vi "AuMT8852B AFH EUT Report Rate.vi"(5 "EUT Reporting Rate (1)":i8=1 min=1 max=30, 7 "Set/Get (Set)":enum16{"Set", "Get"}(ring)=enum."Get", 8 "error in (no error)":errorcluster, 11 "VISA session":refnum<visa-resource-name>) -> (0 "error out":errorcluster, 2 "error code":i32, 3 "VISA session out":refnum<visa-resource-name>, 4 "EUT Reporting Rate out":i8=1 min=1 max=30)   [LabVIEW 2017]
doc: "Anritsu MT8852B Bluetooth Tester\n\nControls the rate, in seconds, at which the EUT generates local assessment reports.\n\nINPUTS\nSet/Get - whether the value is being sent to or retrieved from the instrument.\nEUT Reporting Rate - the rate (1-30 seconds) at which reports are generated.\n\nOUTPUTS\nEUT Reporting Rate out - the current rate at which reports are currently generated."
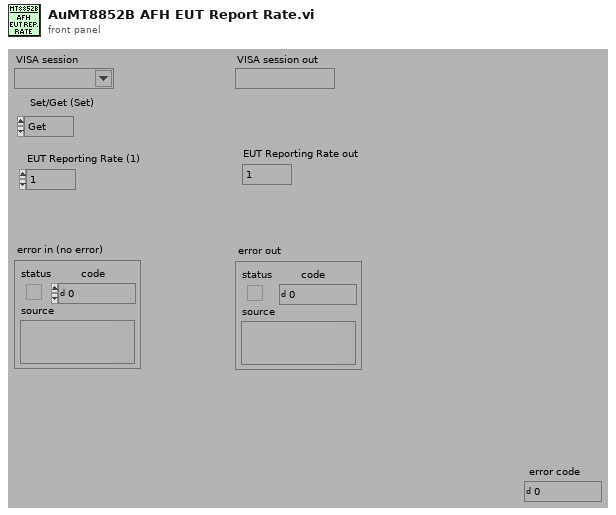
[diagram p1: front panel]
types:
  T1 = enum16{"Simulate", "Range check", "Cache", "Query instrument status"}
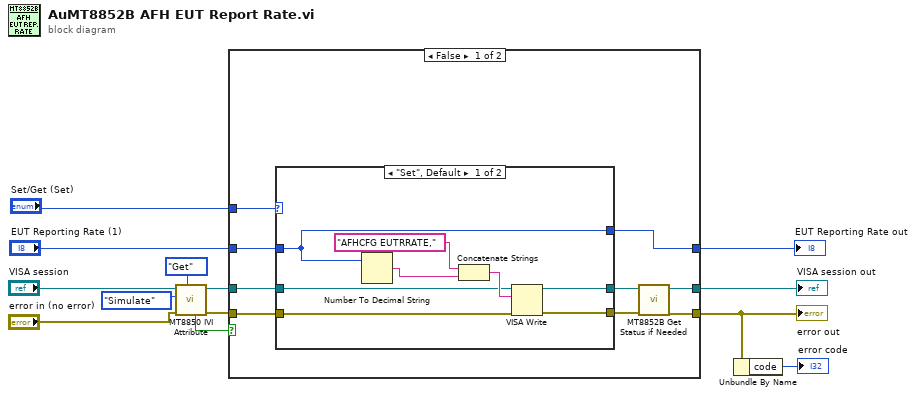
[diagram p0: block diagram]
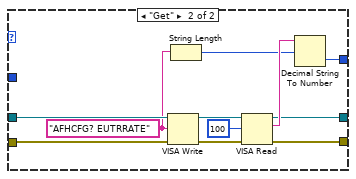
[diagram p2: hidden frame]
diagram:
  n1 = call <instrlib>:"MT8850 IVI Attribute.vi"("Set/Get (Set)"=enum16{"Set", "Get"}."Get", "error in (no error)"="error in (no error)", "Flag (Simulate)"=T1."Simulate", "VISA session"="VISA session") -> ("error out"=w12:errorcluster, "VISA session out"=w13:refnum<visa-resource-name>, "Value out"=w9:bool)  [unwired: 5 in]
  n2 = case shown="False" w9 {
    tunnel: [w18 w44] -> w7
    tunnel: [w19 w43] -> w6
    tunnel: w13 -> [w20 w44]
    tunnel: w12 -> [w21 w43]
    tunnel: [w22 w42] -> w3
    tunnel: "EUT Reporting Rate (1)" -> [w15 w42]
    tunnel: "Set/Get (Set)" -> [w14 _]
    frame False {
      n3 = case shown="\"Set\", Default" w14 {
        tunnel: w15 -> [w24 _]
        tunnel: [w24 w37] -> w22
        tunnel: [w25 w34] -> w16
        tunnel: [w26 w33] -> w17
        tunnel: w21 -> [w28 w36]
        tunnel: w20 -> [w27 w35]
        frame "Set", Default {
          n4 = Number To Decimal String(number=w24) -> (decimal integer string=w23:string)  [unwired: 1 in]
          n5 = Concatenate Strings("AFHCFG EUTRRATE," ("write buffer (\"\")"), w23) -> (w29:string)
          n6 = VISA Write(VISA resource name=w27, write buffer=w29, error in (no error)=w28) -> (VISA resource name out=w26:refnum<visa-resource-name>, error out=w25:errorcluster)  [unwired: 1 out]
        }
        frame "Get" {
          w32 = "AFHCFG? EUTRRATE" ("write buffer (\"\")")
          n7 = VISA Write(VISA resource name=w35, write buffer=w32, error in (no error)=w36) -> (VISA resource name out=w40:refnum<visa-resource-name>, error out=w41:errorcluster)  [unwired: 1 out]
          n8 = String Length(string=w32) -> (length=w31:i32)
          n9 = VISA Read(VISA resource name=w40, byte count=u32 100 ("byte count (0)"), error in (no error)=w41) -> (VISA resource name out=w33:refnum<visa-resource-name>, read buffer=w38:string, error out=w34:errorcluster)  [unwired: 1 out]
          n10 = Decimal String To Number(string=w38, offset=w31) -> (number=w37:i32)  [unwired: 1 in, 1 out]
        }
      }
      n11 = call <instrlib>:"MT8852B Get Status if Needed.vi"("error in (no error)"=w16, "VISA session"=w17) -> ("error out"=w19:errorcluster, "VISA session out"=w18:refnum<visa-resource-name>)  [unwired: 8 in]
    }
    frame True {
    }
  }
  "error out" <- w6
  "VISA session out" <- w7
  "EUT Reporting Rate out" <- w3
  n12 = Unbundle By Name(w6) -> ("code"=→"error code":i32)
